vi "file_version.vi"(4 "custom_path":path, 6 "force_read?":bool, 7 "command":T2=enum."read_config", 8 "error in (no error)":errorcluster, 10 "project_file":path, 11 "version in":T1) -> (0 "error out":errorcluster, 3 "version out":T1)   [LabVIEW 2015, in "lv-builder-default.lvlib"]
doc: "This VI can be used to store the runtime/configuration information for a given project file. The JSON file is stored within application data."
uses:
  lv-builder-default.lvlib
  _controls/version.ctl
  _controls/version_command.ctl
  lv-build/lv-build.lvlib
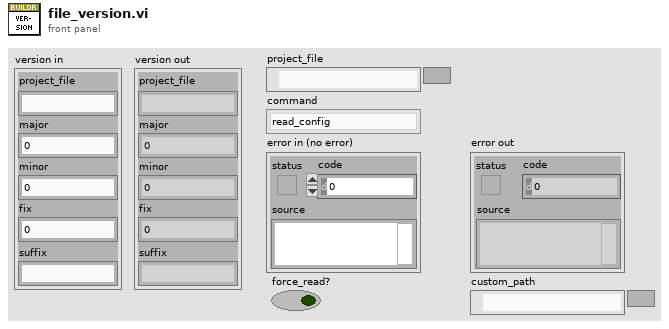
[diagram p1: front panel]
types:
  T1 = typedef "lv-builder-default.lvlib/version.ctl" = cluster{"project_file":string, "major":u32, "minor":u32, "fix":u32, "suffix":string}
  T2 = typedef "lv-builder-default.lvlib/version_command.ctl" = enum16{"<version_command>", "read_config", "write_config", "<null>"}
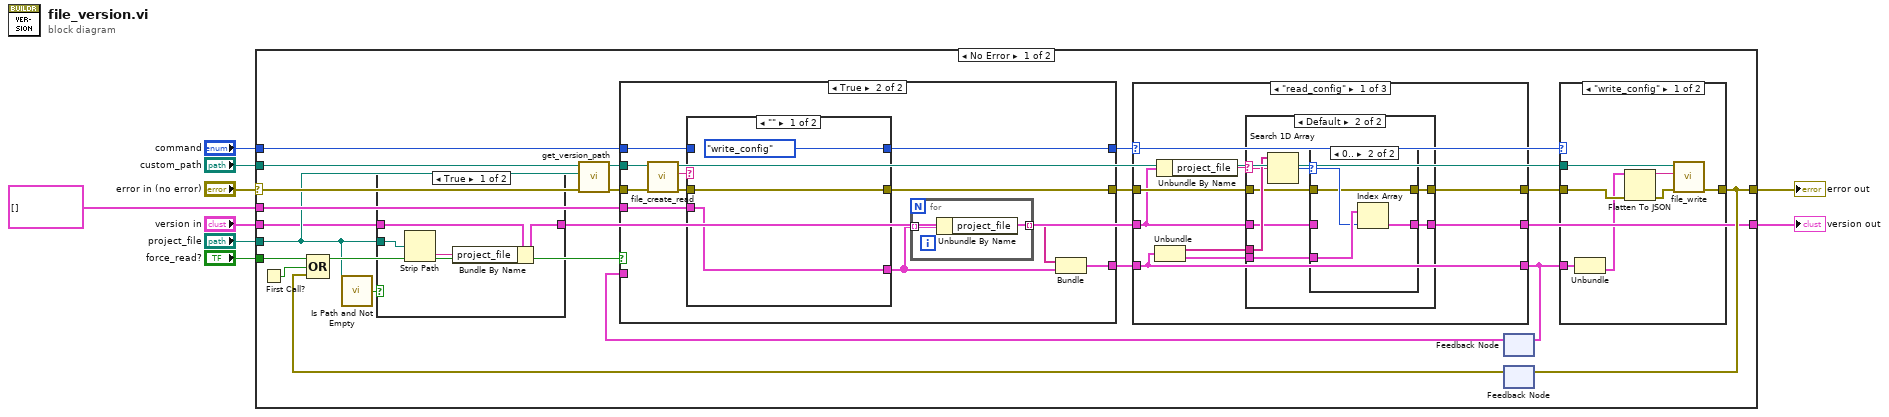
[diagram p0: block diagram]
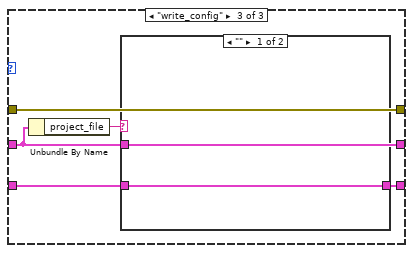
[diagram p6: hidden frame]
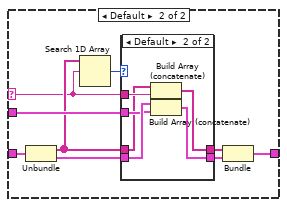
[diagram p7: hidden frame]
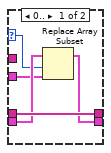
[diagram p8: hidden frame]
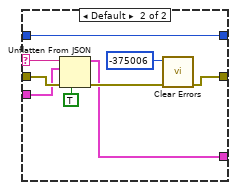
[diagram p10: hidden frame]
diagram:
  n1 = case shown="No Error" "error in (no error)" {
    selector: "error in (no error)" -> [w23 w126]
    tunnel: "command" -> [w25 _]
    tunnel: [w31 w126] -> w6
    tunnel: "version in" -> [w11 _]
    tunnel: "force_read?" -> [w28 _]
    tunnel: T1[] [] -> [w26 _]
    tunnel: [w17 _] -> w1
    tunnel: "project_file" -> [w12 _]
    tunnel: "custom_path" -> [w14 _]
    frame No Error {
      n2 = First Call?() -> (First Call?: T/F=w29:bool)
      n3 = call <vilib>:"Is Path and Not Empty.vi"("path"=w12) -> ("Is Path and Not Empty?"=w13:bool)  [unwired: 4 in]
      n4 = case shown="True" w13 {
        tunnel: w11 -> [w35 w36]
        tunnel: [w34 w36] -> w10
        tunnel: w12 -> [w33 _]
        frame True {
          n5 = Strip Path(path=w33) -> (name=w32:string)  [unwired: 1 out]
          n6 = Bundle By Name(cluster=w35, "project_file"=w32) -> (w34:T1)
        }
        frame False {
        }
      }
      n7 = call "get_version_path.vi"("error in (no error)"=w23, "project_file"=w12, "custom_path"=w14) -> ("error out"=w22:errorcluster, "lv_build_version_path"=w24:path)  [unwired: 7 in]
      n8 = feedback #1() -> (w21:cluster{string[], T1[]})  [unwired: 1 in]
      n9 = feedback #2() -> (w30:errorcluster)  [unwired: 1 in]
      n10 = Compound Arithmetic op=OR(w28, w29, w30) -> (w27:bool)
      n11 = case shown="True" w27 {
        tunnel: w21 -> [w90 _]
        tunnel: w22 -> [w92 w101]
        tunnel: w24 -> [_ w102]
        tunnel: [w92 w99] -> w16
        tunnel: w26 -> [_ w103]
        tunnel: w25 -> [w91 w98]
        tunnel: [w91 w97] -> w18
        tunnel: [w90 w94] -> w19
        frame False {
        }
        frame True {
          n12 = call "file_create_read.vi"("error in (no error)"=w101, "config_path"=w102) -> ("error out"=w100:errorcluster, "string"=w96:string)  [unwired: 8 in]
          n13 = case shown="\"\"" w96 {
            selector: w96 -> [_ w115]
            tunnel: w103 -> [w107 w116]
            tunnel: [w107 w109] -> w95
            tunnel: w100 -> [w108 w117]
            tunnel: [w108 w110] -> w99
            tunnel: w98 -> [_ w114]
            tunnel: [version_command."write_config" ("command") w114] -> w97
            frame "" {
            }
            frame Default {
              n14 = Unflatten From JSON(JSON string=w115, type and defaults=w116, default null elements? (F)=TRUE, error in (no error)=w117) -> (value=w109:T1[], error out=w112:errorcluster)  [unwired: 3 in]
              n15 = call <vilib>:"Clear Errors.vi"("error in (no error)"=w112, "specific error code to clear (0: all)"=-375006) -> ("error out"=w110:errorcluster)  [unwired: 4 in, 1 out]
            }
          }
          n16 = for {
            tunnel: w95 -> [w105] mode=indexing
            tunnel: [w104] -> w93 mode=indexing
            n17 = Unbundle By Name(w105) -> ("project_file"=w104:string)
          }
          n18 = Bundle(w93, w95) -> (w94:cluster{string[], T1[]})  [unwired: 1 in]
        }
      }
      n19 = case shown="\"read_config\"" w18 {
        tunnel: w10 -> [w37 w63 w65]
        tunnel: [w44 w62 w68] -> w20
        tunnel: w19 -> [w44 w62 w66]
        tunnel: [w40 w63 w65] -> w17
        tunnel: w16 -> [w39 w61 w64]
        tunnel: [w38 w61 w64] -> w15
        frame "read_config" {
          n20 = Unbundle(w44) -> (w43:string[], w42:T1[])
          n21 = Unbundle By Name(w37) -> ("project_file"=w41:string)
          n22 = case shown="Default" w41 {
            selector: w41 -> [_ w51]
            tunnel: w43 -> [_ w54]
            tunnel: w42 -> [_ w53]
            tunnel: [w45 w50] -> w40
            tunnel: w39 -> [w46 w49]
            tunnel: [w46 w48] -> w38
            tunnel: w37 -> [w45 w47]
            frame "" {
            }
            frame Default {
              n23 = Search 1D Array(1D array=w54, element=w51) -> (index of element=w52:i32)  [unwired: 1 in]
              n24 = case shown="0.." w52 {
                selector: w52 -> [_ w59]
                tunnel: w53 -> [_ w60]
                tunnel: [w55 w58] -> w50
                tunnel: w49 -> [w56 w57]
                tunnel: [w56 w57] -> w48
                tunnel: w47 -> [w55 _]
                frame Default {
                }
                frame 0.. {
                  n25 = Index Array(array=w60, index=w59) -> (element=w58:T1)
                }
              }
            }
          }
        }
        frame Default {
        }
        frame "write_config" {
          n26 = Unbundle By Name(w65) -> ("project_file"=w67:string)
          n27 = case shown="\"\"" w67 {
            selector: w67 -> [_ w70]
            tunnel: [w69 w76] -> w68
            tunnel: w65 -> [_ w74]
            tunnel: w66 -> [w69 w72]
            frame "" {
            }
            frame Default {
              n28 = Unbundle(w72) -> (w71:string[], w73:T1[])
              n29 = Search 1D Array(1D array=w71, element=w70) -> (index of element=w78:i32)  [unwired: 1 in]
              n30 = case shown="Default" w78 {
                selector: w78 -> [w79 _]
                tunnel: w73 -> [w82 w88]
                tunnel: [w81 w86] -> w77
                tunnel: w71 -> [w83 w84]
                tunnel: [w83 w85] -> w75
                tunnel: w74 -> [w80 w87]
                tunnel: w70 -> [_ w89]
                frame 0.. {
                  n31 = Replace Array Subset(array=w82, new element=w80, index=w79) -> (w81:T1[])
                }
                frame Default {
                  n32 = Build Array (concatenate)(w84, w89) -> (w85:string[])
                  n33 = Build Array (concatenate)(w88, w87) -> (w86:T1[])
                }
              }
              n34 = Bundle(w75, w77) -> (w76:cluster{string[], T1[]})  [unwired: 1 in]
            }
          }
        }
      }
      n35 = feedback-in #1(w20) -> ()
      n36 = case shown="\"write_config\"" w18 {
        tunnel: w20 -> [w119 _]
        tunnel: w15 -> [w122 w125]
        tunnel: [w120 w125] -> w31
        tunnel: w24 -> [w121 _]
        frame "write_config" {
          n37 = Unbundle(w119) -> (w118:T1[])  [unwired: 1 out]
          n38 = Flatten To JSON(anything=w118, error in (no error)=w122) -> (JSON string=w124:string, 11:w123:errorcluster)  [unwired: 1 in]
          n39 = call "file_write.vi"("error in (no error)"=w123, "string"=w124, "config_path"=w121) -> ("error out"=w120:errorcluster)  [unwired: 8 in]
        }
        frame Default {
        }
      }
      n40 = feedback-in #2(w31) -> ()
    }
    frame Error {
      # "If an error is wired in, be sure to skip over functionality to preserve the original error"
    }
  }
  "error out" <- w6
  "version out" <- w1
